vi "G# - PerformanceComparision.vi"() -> ()   [LabVIEW 2020]
doc: "Data Value Reference Approach\n\nThis example demonstates the difference between using the memory pointer to access the attributes when havin a large amount of data in the attributes.\n\nOpen the \"ReadAttributeSlow.vi\" and the \"ReadAttributeFast.vi\" to compare implementations.\n\nBy using the G# Debugger found in Tools->G# Debugger a text log can be followed showing how the objects were created and destroyed."
uses:
  TestClass_class/TestClass.lvclass
  <vilib>/addons/_AddQ/G#Object/G#Object.lvclass
panel:
  out "# of objects killed":i32
  out "OK":bool
  in  "error in (no error)":errorcluster
  out "FastAccess (ms)":u32
  out "Slow Access (ms)":u32
  out "error out":errorcluster
  # "Data Value Reference Approach\n\nThis example demonstates the difference between using the memory pointer to access the attributes when havin a large amount of data in the attributes.\n\nOpen the \"ReadAttributeSlow.vi\" and the \"ReadAttributeFast.vi\" to compare implementations.\n\nBy using the G# Debugger found in Tools->G# Debugger a text log can be followed showing how the objects were created and destroyed."
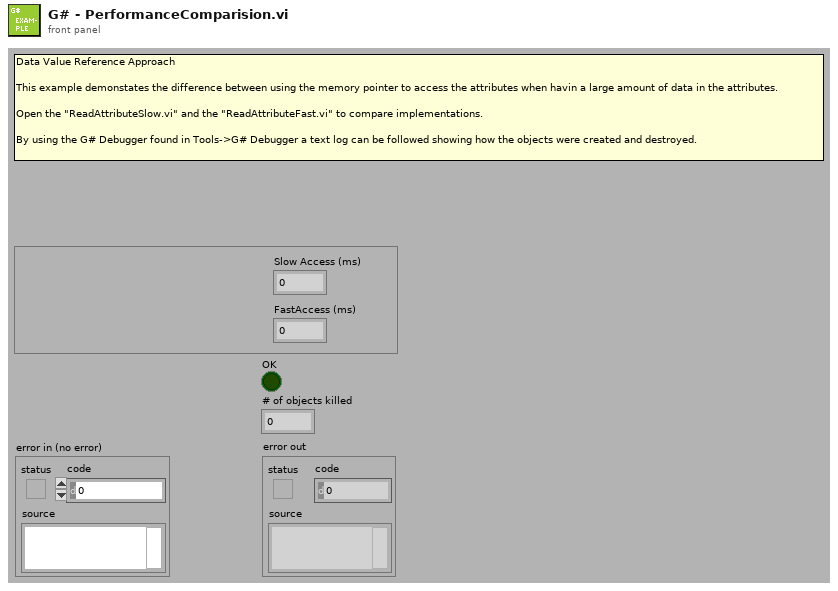
[diagram p1: front panel]
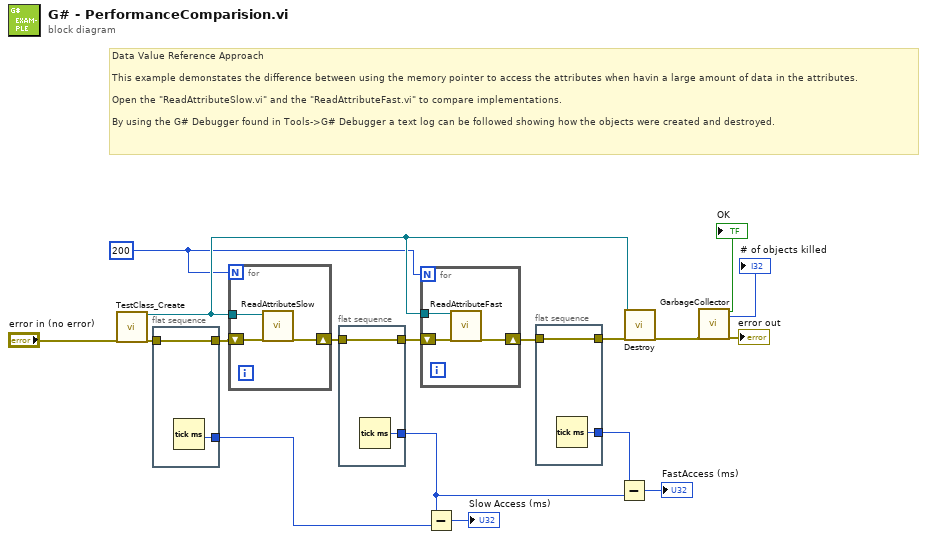
[diagram p0: block diagram]
diagram:
  w14 = 200
  # "Data Value Reference Approach\n\nThis example demonstates the difference between using the memory pointer to access the attributes when havin a large amount of data in the attributes.\n\nOpen the \"ReadAttributeSlow.vi\" and the \"ReadAttributeFast.vi\" to compare implementations.\n\nBy using the G# Debugger found in Tools->G# Debugger a text log can be followed showing how the objects were created and destroyed."
  n1 = call "TestClass_Create.vi"("error in (no error)"="error in (no error)") -> ("reference out"=w15:refnum<class "TestClass.lvclass">, "error out"=w13:errorcluster)  [unwired: 17 in]
  n2 = flat-sequence {
    tunnel: w13 -> [w20]
    tunnel: [w20] -> w12
    tunnel: [w19] -> w7
    frame #0 {
      n3 = Tick Count (ms)() -> (millisecond timer value=w19:u32)
    }
  }
  n4 = for {
    N: w14 -> [_]
    tunnel: w15 -> [w22]
    shift-right: [w21] -> w11
    shift-left: w12 -> [w23]
    n5 = call-dynamic "ReadAttributeSlow.vi"("reference in"=w22, "error in (no error)"=w23) -> ("error out"=w21:errorcluster)  [unwired: 15 in, 2 out]
  }
  n6 = flat-sequence {
    tunnel: w11 -> [w25]
    tunnel: [w25] -> w10
    tunnel: [w24] -> w5
    frame #0 {
      n7 = Tick Count (ms)() -> (millisecond timer value=w24:u32)
    }
  }
  n8 = for {
    N: w14 -> [_]
    shift-right: [w27] -> w9
    shift-left: w10 -> [w28]
    tunnel: w15 -> [w26]
    n9 = call-dynamic "ReadAttributeFast.vi"("reference in"=w26, "error in (no error)"=w28) -> ("error out"=w27:errorcluster)  [unwired: 15 in, 2 out]
  }
  n10 = Subtract(x=w5, y=w7) -> (x-y=→"Slow Access (ms)":u32)
  n11 = flat-sequence {
    tunnel: w9 -> [w30]
    tunnel: [w30] -> w8
    tunnel: [w29] -> w6
    frame #0 {
      n12 = Tick Count (ms)() -> (millisecond timer value=w29:u32)
    }
  }
  n13 = Subtract(x=w6, y=w5) -> (x-y=→"FastAccess (ms)":u32)
  n14 = call-dynamic "Destroy.vi"("reference in"=w15, "error in (no error)"=w8) -> ("error out"=w18:errorcluster)  [unwired: 16 in, 1 out]
  n15 = call <vilib>:"GarbageCollector.vi"("error in (no error)"=w18) -> ("OK"=→"OK":bool, "# of objects killed"=→"# of objects killed":i32, "error out"=→"error out":errorcluster)  [unwired: 16 in]
